vi "Get Type.vi"() -> ()   [LabVIEW 2015]
doc: "<b> </b> <b> </b>\n©2016 Q Software Innovations, LLC (QSI)\nwritten by Quentin Alldredge\nproduced in LabVIEW 2015"
uses:
  Project Manipulation Scripts/Project Manipulation Scripts.lvlib
panel:
  out "Array":T1(array[cluster])
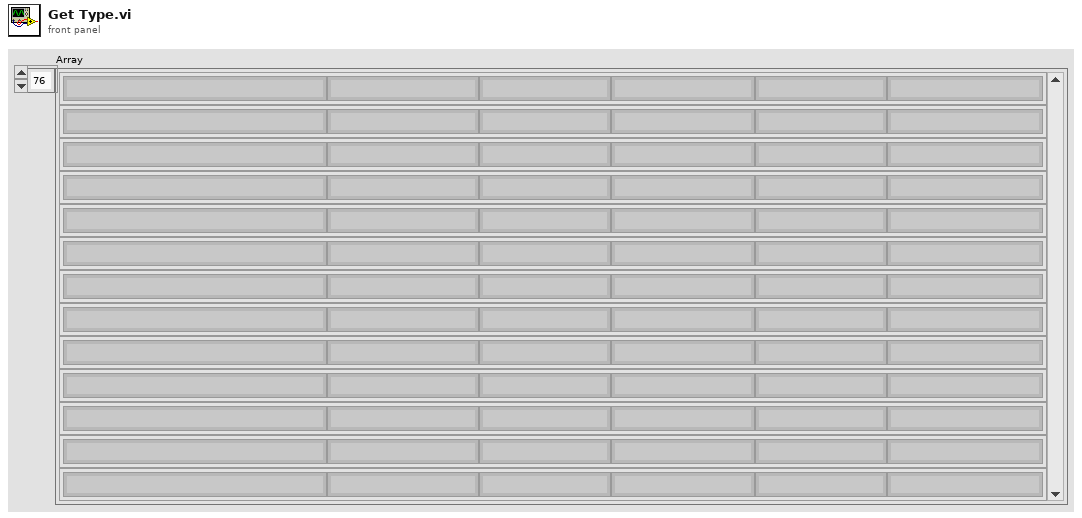
[diagram p1: front panel]
types:
  T1 = cluster{"Display Name":string, "Type String":string, "Library Item Type String":string, string, "output string":string, "output string":string}[]
  T2 = enum32{"invalid VI type", "Standard VI", "Control VI", "Global VI", "Polymorphic VI", "Configuration VI", "SubSystem", "Facade VI", "Method VI", "Statechart Diagram VI"}
  T3 = cluster{"Display Name":string, "Type String":string, "Library Item Type String":string, string, "output string":string, "output string":string}
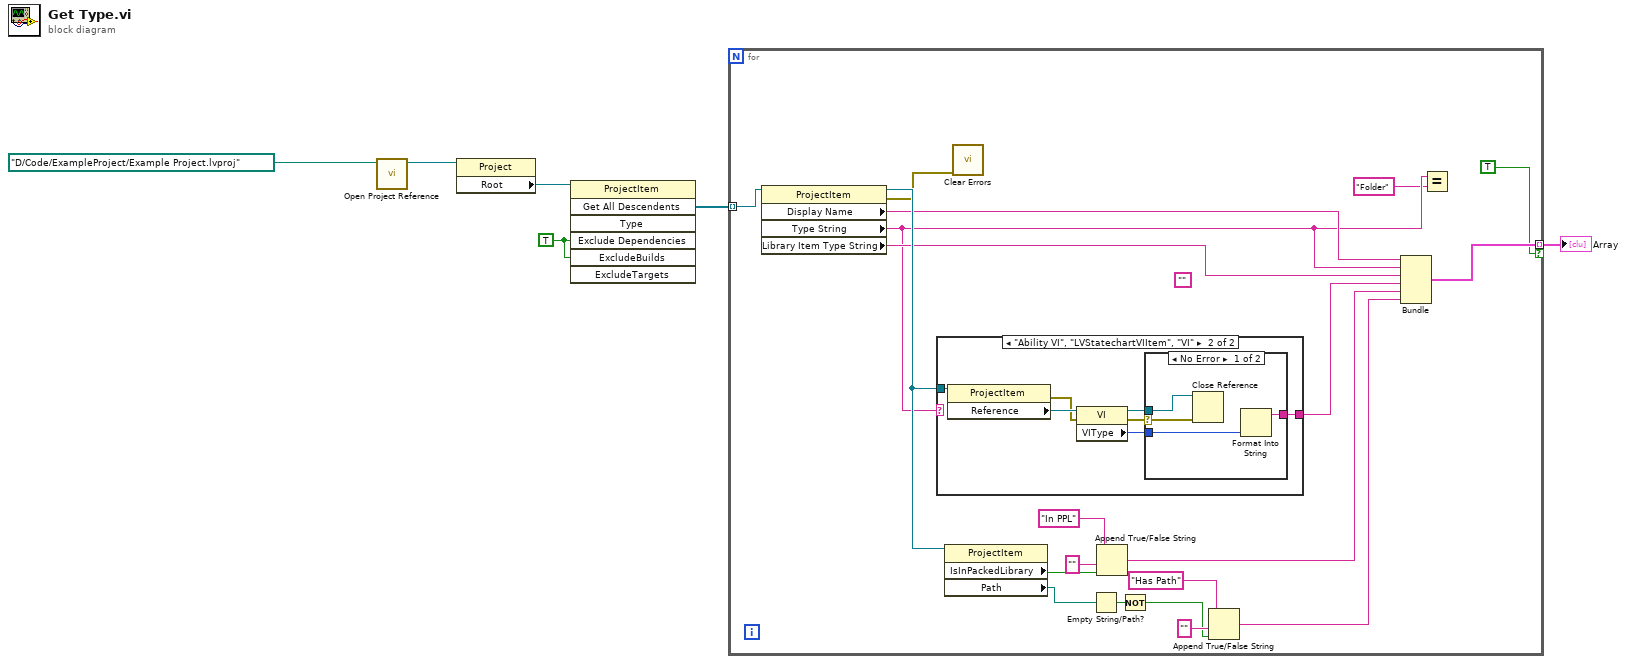
[diagram p0: block diagram]
diagram:
  w1 = TRUE ("ExcludeDependencies")
  n1 = call "Open Project Reference.vi"("Project Path"=path "D:/Code/ExampleProject/Example Project.lvproj" ("Path")) -> ("Project out"=w5:refnum<vi>)  [unwired: 10 in]
  n2 = property class="Project"(reference=w5) -> ("Root"=w4:refnum<vi>)  [unwired: 1 in, 2 out]
  n3 = invoke class="ProjectItem" method="Get All Descendents"(reference=w4, "Exclude Dependencies"=w1, "ExcludeBuilds"=w1) -> ("All Descendents"=w3:refnum<vi>[])  [unwired: 4 in, 6 out]
  n4 = for {
    tunnel: w3 -> [w26] mode=indexing
    tunnel: [w13] -> w2 mode=indexing if=TRUE
    (unwired) ""
    n5 = property class="ProjectItem"(reference=w26) -> (reference out=w24:refnum<vi>, error out=w11:errorcluster, "Display Name"=w12:string, "Type String"=w9:string, "Library Item Type String"=w10:string)  [unwired: 1 in]
    n6 = case shown="\"Ability VI\", \"LVStatechartVIItem\", \"VI\"" w9 {
      tunnel: [_ w31] -> w25
      tunnel: w24 -> [_ w27]
      frame Default {
      }
      frame "Ability VI", "LVStatechartVIItem", "VI" {
        n7 = property class="ProjectItem"(reference=w27) -> (error out=w30:errorcluster, "Reference"=w33:refnum<vi>)  [unwired: 1 in, 1 out]
        n8 = property class="VI"(reference=w33, error in=w30) -> (reference out=w28:refnum<vi>, error out=w29:errorcluster, "VIType"=w32:T2)
        n9 = case shown="No Error" w29 {
          selector: w29 -> [w34 _]
          tunnel: w32 -> [w37 _]
          tunnel: [w36 _] -> w31
          tunnel: w28 -> [w35 _]
          frame No Error {
            n10 = Close Reference(reference=w35, error in (no error)=w34) -> ()  [unwired: 1 out]
            n11 = Format Into String(w37) -> (resulting string=w36:string)  [unwired: 3 in, 1 out]
          }
          frame Error {
          }
        }
      }
    }
    n12 = property class="ProjectItem"(reference=w24) -> ("IsInPackedLibrary"=w23:bool, "Path"=w19:path)  [unwired: 1 in, 2 out]
    n13 = call <vilib>:"Clear Errors.vi"("error in (no error)"=w11) -> ()  [unwired: 5 in, 2 out]
    n14 = Empty String/Path?(string/path=w19) -> (empty?=w16:bool)
    n15 = Append True/False String(1:w23, 2:"" ("false string"), 3:"In PPL" ("true string")) -> (0:w20:string)  [unwired: 1 in]
    n16 = Not(x=w16) -> (.not. x?=w14:bool)
    n17 = Append True/False String(1:w14, 2:"" ("false string"), 3:"Has Path" ("true string")) -> (0:w15:string)  [unwired: 1 in]
    n18 = Bundle("Display Name"=w12, "Type String"=w9, "Library Item Type String"=w10, w25, "output string"=w20, "output string"=w15) -> (w13:T3)  [unwired: 1 in]
    n19 = Equal?(x=w9, y="Folder") -> ()  [unwired: 1 out]
  }
  "Array" <- w2
